vi "DSF.Engine.Status.Framework.Performance.Get Rx Duration.vi"(8 "error in (no error)":errorcluster, 11 "Framework Performance in":refnum<class "DSF.Engine.Status.Framework.Performance.lvclass">) -> (0 "error out":errorcluster, 2 "rx duration":u32 format="%d us", 3 "Framework Performance out":refnum<class "DSF.Engine.Status.Framework.Performance.lvclass">)   [LabVIEW 2017, in "DSF.Engine.lvlib" / "DSF.Engine.Status.Framework.Performance.lvclass"]
uses:
  DSF.Engine.Status.Framework.Performance.lvclass
  DSF.Engine.Status.Framework.Performance.lvclass/DSF.Engine.Status.Framework.Performance.ctl
  Built/Memory/Memory Manager.lvlibp/1abvi3w/vi.lib/National Instruments/Memory Manager/Classes/Pointer/Memory.Pointer.Read.0D.U32.vi
  Built/Memory/Memory Manager.lvlibp/1abvi3w/vi.lib/National Instruments/Memory Manager/Classes/Pointer/Memory.Pointer.lvclass
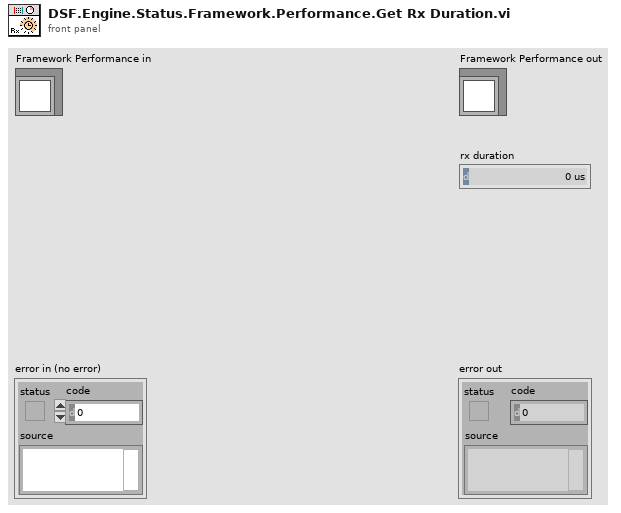
[diagram p1: front panel]
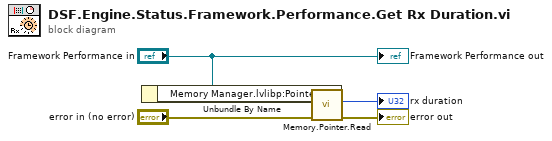
[diagram p0: block diagram]
diagram:
  n1 = Unbundle By Name("Framework Performance in") -> ("Memory Manager.lvlibp:Pointer 2"=w4:refnum<class "Memory.Pointer.lvclass">)
  n2 = call-poly "Memory.Pointer.Read.vi"("error in (no error)"="error in (no error)", "Pointer in"=w4) -> ("error out"=→"error out":errorcluster, "value out"=→"rx duration":u32)  [unwired: 6 in, 2 out]
  "Framework Performance out" <- "Framework Performance in"
